vi "AutoCommands.vi"() -> ()   [LabVIEW 2019]
panel:
  out "DriveTurn":dbl
  out "PrimeShooterSpeed(rpm)":dbl
  out "PrimeShooter":bool
  out "DriveSpeed":dbl
  out "Intake":bool
  out "Shoot":bool
  out "Aim":bool
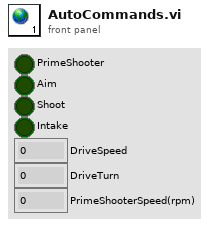
[diagram p1: front panel]
diagram:
